vi "GetGrowInfo.vi"(0 "XRef":T16, 1 "State In":T6) -> (14 "Grow Info":T2, 15 "Fatal Error Out":T1)   [LabVIEW 2020, in "Parallel Diagram Block.xnode"]
uses:
  Parallel Diagram Block.xnode
  <vilib>/XNodeSupport/XNodeXNodeRef.ctl
  State.ctl
  Parallel Block/Type Descriptor.ctl
  Parallel Block/Direction.ctl
  Parallel Block/Value Type.ctl
  Parallel Block/Terminal Mode.ctl
  Parallel Block/Terminal Type.ctl
  Parallel Block/Type Mode.ctl
  Parallel Block/Value Mode.ctl
  <vilib>/picture/picture.llb/imagedata.ctl
  Parallel Block/Manager Node.ctl
  <vilib>/XNodeSupport/XNodeGrowInfo.ctl
  <vilib>/XNodeSupport/XNodeBounds.ctl
  <vilib>/XNodeSupport/XNodeInt.ctl
  <vilib>/XNodeSupport/XNodeBool.ctl
  <vilib>/XNodeSupport/XNodeErrorCluster.ctl
  <vilib>/XNodeSupport/NI_XNodeSupport.lvlib
  Parallel Block/Parallel Block.lvlib
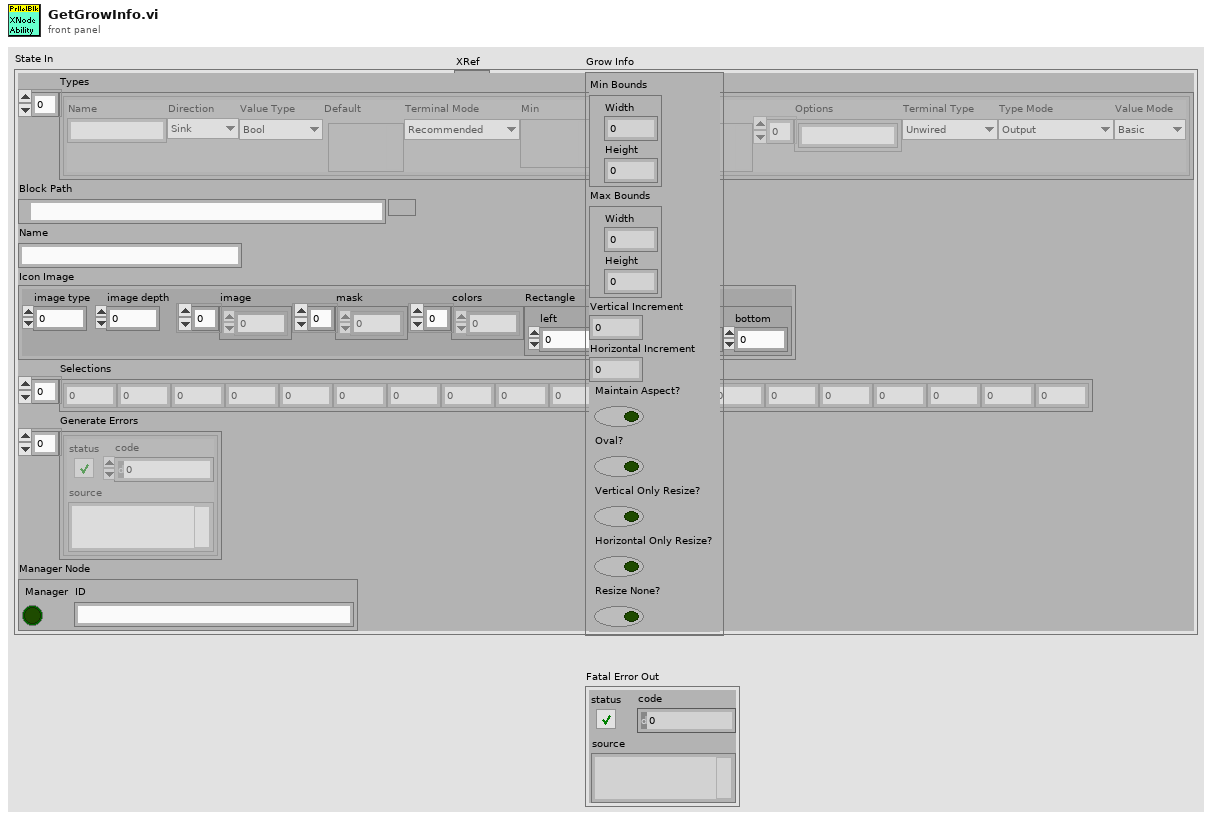
[diagram p1: front panel]
types:
  T1 = typedef "NI_XNodeSupport.lvlib/XNodeErrorCluster.ctl" = errorcluster
  T2 = typedef "NI_XNodeSupport.lvlib/XNodeGrowInfo.ctl" = cluster{"Min Bounds":T3, "Max Bounds":T3, "Vertical Increment":T4, "Horizontal Increment":T4, "Maintain Aspect?":T5, "Oval?":T5, "Vertical Only Resize?":T5, "Horizontal Only Resize?":T5, "Resize None?":T5}
  T3 = typedef "NI_XNodeSupport.lvlib/XNodeBounds.ctl" = cluster{"Width":T4, "Height":T4}
  T4 = typedef "NI_XNodeSupport.lvlib/XNodeInt.ctl" = i32
  T5 = typedef "NI_XNodeSupport.lvlib/XNodeBool.ctl" = bool
  T6 = typedef "Parallel Diagram Block.xnode/State.ctl" = cluster{"Types":T7[], "Block Path":path, "Name":string, "Icon Image":T14, "Selections":i32[], "Generate Errors":errorcluster[], "Manager Node":T15}
  T7 = typedef "Parallel Block.lvlib/Type Descriptor.ctl" = cluster{"Name":string, "Direction":T8, "Value Type":T9, "Default":variant, "Terminal Mode":T10, "Min":variant, "Max":variant, "Step":variant, "Options":string[], "Terminal Type":T11, "Type Mode":T12, "Value Mode":T13}
  T8 = typedef "Parallel Block.lvlib/Direction.ctl" = enum16{"Sink", "Source"}
  T9 = typedef "Parallel Block.lvlib/Value Type.ctl" = enum16{"Unknown", "Bool", "U8", "U16", "U32", "U64", "I8", "I16", "I32", "I64", "SGL", "DBL", "CSG", "CDB", "CDBWfm", "String", "DBLWfm"}
  T10 = typedef "Parallel Block.lvlib/Terminal Mode.ctl" = enum16{"Recommended", "Required", "None"}
  T11 = typedef "Parallel Block.lvlib/Terminal Type.ctl" = enum16{"Unwired", "BadType", "Connection", "Value", "Control Ref", "BadRefType"}
  T12 = typedef "Parallel Block.lvlib/Type Mode.ctl" = enum16{"Output", "Single - Strict", "Single - Coerced", "Stream"}
  T13 = typedef "Parallel Block.lvlib/Value Mode.ctl" = enum16{"Basic", "Range", "Select"}
  T14 = typedef "imagedata.ctl" = cluster{"image type":i32, "image depth":i32, "image":u8[], "mask":u8[], "colors":u32[], "Rectangle":cluster{"left":i16, "top":i16, "right":i16, "bottom":i16}}
  T15 = typedef "Parallel Block.lvlib/Manager Node.ctl" = cluster{"Manager":bool, "ID":string}
  T16 = typedef "NI_XNodeSupport.lvlib/XNodeXNodeRef.ctl" = refnum<vi>
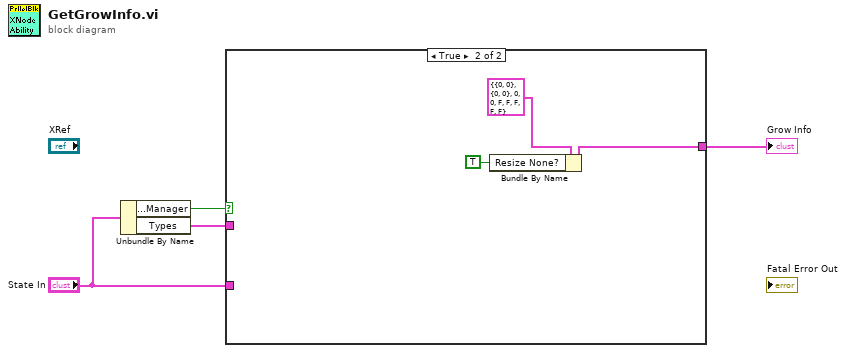
[diagram p0: block diagram]
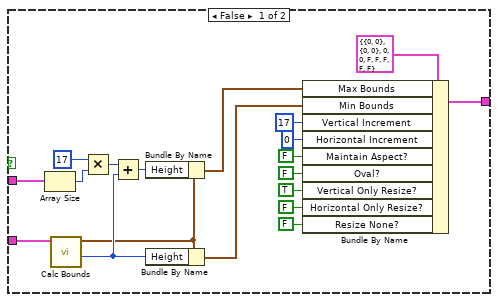
[diagram p2: hidden frame]
diagram:
  n1 = Unbundle By Name("State In") -> ("Manager Node.Manager"=w1:bool, "Types"=w2:T7[])
  n2 = case shown="True" w1 {
    tunnel: [w22 w25] -> w4
    tunnel: "State In" -> [w14 _]
    tunnel: w2 -> [w13 _]
    frame False {
      n3 = Array Size(array=w13) -> (size(s)=w12:i32)
      n4 = call "Calc Bounds.vi"("State"=w14) -> ("Collapsed"=w9:i32, "Text Bounds"=w6:T3)  [unwired: 4 in, 5 out]
      n5 = Multiply(x=17, y=w12) -> (x*y=w10:i32)
      n6 = Add(x=w10, y=w9) -> (x+y=w5:i32)
      n7 = Bundle By Name(cluster=w6, "Height"=w5) -> (w7:T3)
      n8 = Bundle By Name(cluster=w6, "Height"=w9) -> (w8:T3)
      n9 = Bundle By Name(cluster=T2 {"Min Bounds"={"Width"=0, "Height"=0}, "Max Bounds"={"Width"=0, "Height"=0}, "Vertical Increment"=0, "Horizontal Increment"=0, "Maintain Aspect?"=FALSE, "Oval?"=FALSE, "Vertical Only Resize?"=FALSE, "Horizontal Only Resize?"=FALSE, "Resize None?"=FALSE} ("Grow Info"), "Max Bounds"=w7, "Min Bounds"=w8, "Vertical Increment"=T4 17, "Horizontal Increment"=T4 0, "Maintain Aspect?"=T5 FALSE, "Oval?"=T5 FALSE, "Vertical Only Resize?"=T5 TRUE, "Horizontal Only Resize?"=T5 FALSE, "Resize None?"=T5 FALSE) -> (w22:T2)
    }
    frame True {
      n10 = Bundle By Name(cluster=T2 {"Min Bounds"={"Width"=0, "Height"=0}, "Max Bounds"={"Width"=0, "Height"=0}, "Vertical Increment"=0, "Horizontal Increment"=0, "Maintain Aspect?"=FALSE, "Oval?"=FALSE, "Vertical Only Resize?"=FALSE, "Horizontal Only Resize?"=FALSE, "Resize None?"=FALSE} ("Grow Info"), "Resize None?"=T5 TRUE) -> (w25:T2)
    }
  }
  "Grow Info" <- w4
